vi "Untitled 2.vi"() -> ()   [LabVIEW 2015]
uses:
  State_Enum.ctl
panel:
  in  "Menu":T1
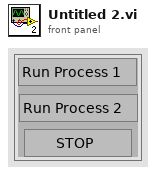
[diagram p1: front panel]
types:
  T1 = cluster{"Process 1":bool, "Process 2":bool, "stop 2":bool}
  T2 = typedef "State_Enum.ctl" = enum32{"Idle", "Process 1", "Process 2", "Stop"}
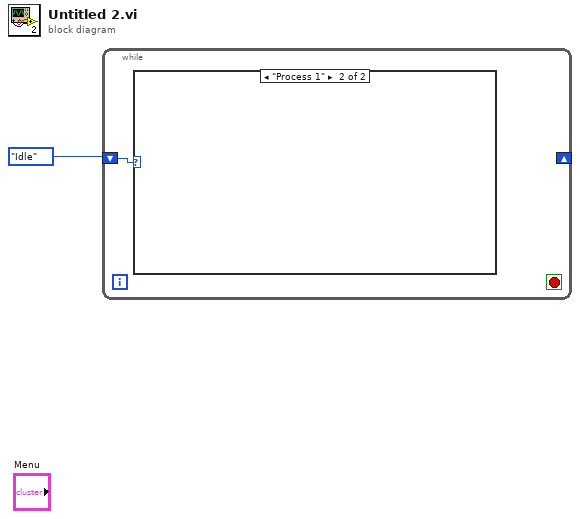
[diagram p0: block diagram]
diagram:
  n1 = while {
    shift-right: _ -> [_]
    shift-left: State_Enum."Idle" ("State Enum") -> [w2]
    stop <- _ stop-if-true
    n2 = case shown="\"Process 1\"" w2 {
      frame "Idle", Default {
      }
      frame "Process 1" {
      }
    }
  }
